vi "Read Name.vi"(8 "error in (no error)":errorcluster, 11 "Topic":refnum<class "Topic.lvclass">) -> (0 "error out":errorcluster, 2 "Name":string, 3 "Topic out":refnum<class "Topic.lvclass">)   [LabVIEW 2015, in "NI_AWS_SNS.lvlib" / "Topic.lvclass"]
uses:
  Topic.lvclass
  Core/ARN/ARN.lvclass/ARN.ctl
  Core/ARN/Read ARN.vi
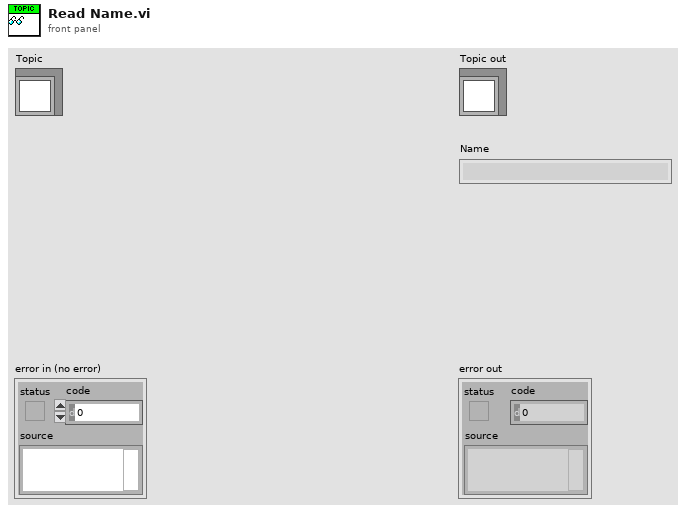
[diagram p1: front panel]
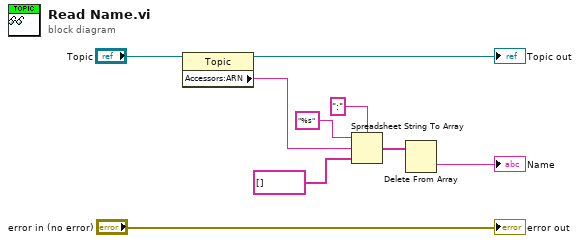
[diagram p0: block diagram]
diagram:
  n1 = property class="Topic"(reference="Topic") -> (reference out=→"Topic out":refnum<class "Topic.lvclass">, "Accessors:ARN"=w1:string)  [unwired: 1 in, 1 out]
  n2 = Spreadsheet String To Array(delimiter (Tab)=":", format string="%s", spreadsheet string=w1, array type (2D Dbl)=string[] []) -> (array=w7:string[])
  n3 = Delete From Array(array=w7) -> (deleted portion=→"Name":string)  [unwired: 2 in, 1 out]
  "error out" <- "error in (no error)"
